vi "Restart.vi"(8 "error in (no error)":errorcluster, 11 "Snake in":refnum<class "SnakeGame.lvclass">) -> (0 "error out":errorcluster, 3 "Snake out":refnum<class "SnakeGame.lvclass">)   [LabVIEW 2019, in "RT_Game.lvlib" / "SnakeGame.lvclass"]
uses:
  SnakeGame.lvclass
  C:/Users/FreshBob/Dropbox/VIs/myRIO_GameConsole/RT/RT_Game/Game/Game.lvclass
  Game/Game.lvclass/Game.ctl
  Game/Game.lvclass
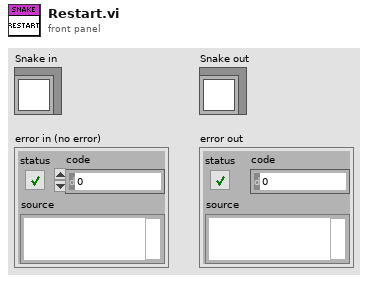
[diagram p1: front panel]
types:
  T1 = cluster{"Controls_1":cluster{"DirectionX":i8, "DirectionY":i8, "Button1":bool, "Button2":bool}, "Controls_2":cluster{"DirectionX":i8, "DirectionY":i8, "Button1":bool, "Button2":bool}, "SystemButton":bool}
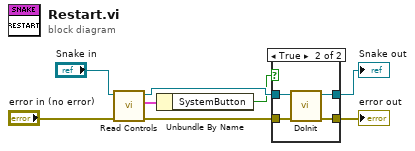
[diagram p0: block diagram]
diagram:
  n1 = call "Read Controls.vi"("error in (no error)"="error in (no error)", "Game in"="Snake in") -> ("error out"=w5:errorcluster, "Controls"=w2:T1, "Game out"=w3:refnum<class "SnakeGame.lvclass">)  [unwired: 7 in]
  n2 = Unbundle By Name(w2) -> ("SystemButton"=w1:bool)
  n3 = case shown="True" w1 {
    tunnel: [w9 w14] -> w7
    tunnel: w3 -> [w10 w13]
    tunnel: [w10 w12] -> w6
    tunnel: w5 -> [w9 w11]
    frame False {
    }
    frame True {
      n4 = call-dynamic "DoInit.vi"("error in (no error)"=w11, "Snake in"=w13) -> ("error out"=w14:errorcluster, "Snake out"=w12:refnum<class "SnakeGame.lvclass">)  [unwired: 8 in]
    }
  }
  "Snake out" <- w6
  "error out" <- w7
